vi "2D curvature tensor algebra.vi"(7 "2D tensor":T2, 9 "2D curvature Matrix IN":T1, 11 "curvature tensor IN":T3={"curvature Matrix"=[[3.0, 1.0], [1.0, 4.0]], "eigenvs"=[4.618033988749895, 2.381966011250105], "Eigenvectors"=[[-0.8506508083520399+0.0i, -0.5257311121191335+0.0i], [0.5257311121191335+0.0i, -0.8506508083520399+0.0i]], "theta (rad)"=0.5535743588970453, "theta (deg)"=31.717474411461012, "Δs"=[4.618033988749895, 2.381966011250105], "δG/G"=0.5535743588970453, "δs"=[4.618033988749895, 2.381966011250105], "inverse Matrix"=[[3.0, 1.0], [1.0, 4.0]], "noise T"=0.5535743588970453, "errors"={}} {"noise T" format="%#_3p"; "inverse Matrix" format="%#_3p"; "δs" format="%#_2p"; "δG/G" format="%#_3p"; "Δs" format="%#_3p"; "theta (deg)" format="%#_3p"; "curvature Matrix" format="%#_3p"; "eigenvs" format="%#_3p"; "Eigenvectors" format="%#_3p"; "theta (rad)" format="%#_3p"}) -> (1 "2D curvature Matrix OUT":T1, 3 "curvature tensor OUT":T3={"curvature Matrix"=[[3.0, 1.0], [1.0, 4.0]], "eigenvs"=[4.618033988749895, 2.381966011250105], "Eigenvectors"=[[-0.8506508083520399+0.0i, -0.5257311121191335+0.0i], [0.5257311121191335+0.0i, -0.8506508083520399+0.0i]], "theta (rad)"=0.5535743588970453, "theta (deg)"=31.717474411461012, "Δs"=[4.618033988749895, 2.381966011250105], "δG/G"=0.5535743588970453, "δs"=[4.618033988749895, 2.381966011250105], "inverse Matrix"=[[3.0, 1.0], [1.0, 4.0]], "noise T"=0.5535743588970453, "errors"={}} {"noise T" format="%#_3p"; "inverse Matrix" format="%#_3p"; "δs" format="%#_2p"; "δG/G" format="%#_3p"; "Δs" format="%#_3p"; "theta (deg)" format="%#_3p"; "curvature Matrix" format="%#_3p"; "eigenvs" format="%#_3p"; "Eigenvectors" format="%#_3p"; "theta (rad)" format="%#_3p"})   [LabVIEW 2020]
uses:
  2D curvature tensor.ctl
  <vilib>/Analysis/Matrix/Datatypes/RealMatrix.ctl
  <vilib>/Analysis/Matrix/Datatypes/ComplexMatrix.ctl
  3-lorentzian-parameters.ctl
  2D curvature tensor actions.ctl
  array of vectors -- algebra.ctl
  <vilib>/Analysis/baseanly.llb/Real Inverse Matrix.vi
  <vilib>/Analysis/7linalg.llb/Real Eigenvalues and Vectors.vi
  <vilib>/Analysis/NI_AALPro.lvlib
  <vilib>/Analysis/NI_AALBase.lvlib
  <vilib>/Analysis/Matrix/NI_Matrix.lvlib
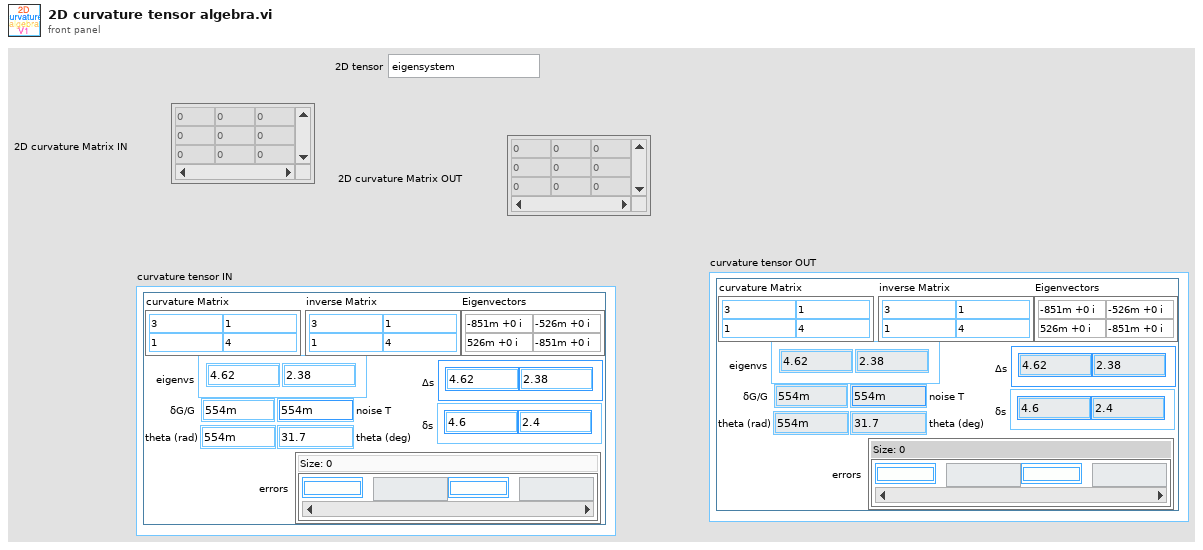
[diagram p1: front panel]
types:
  T1 = typedef "NI_Matrix.lvlib/RealMatrix.ctl" = dbl[][]
  T2 = typedef "2D curvature tensor actions.ctl" = enum16{"eigensystem", "sigma", "set matrix", "inverse"}
  T3 = typedef "2D curvature tensor.ctl" = cluster{"curvature Matrix":T1, "eigenvs":dbl[], "Eigenvectors":T4, "theta (rad)":dbl, "theta (deg)":dbl, "Δs":dbl[], "δG/G":dbl, "δs":dbl[], "inverse Matrix":T1, "noise T":dbl, "errors":map{T5, dbl}}
  T4 = typedef "NI_Matrix.lvlib/ComplexMatrix.ctl" = cdb[][]
  T5 = typedef "3-lorentzian-parameters.ctl" = enum16{"ζ", "τ1", "τS", "τN", "τC", "κ0", "m1", "m2", "m3", "T (K)", "B (T)", "θ (deg)", "side (S|R)", "set of (B|T)", "Re(offset)", "Im(offset)", "στ1", "στ1-", "στ1+", "στS", "στS-", "στS+"}
  T6 = typedef "array of vectors -- algebra.ctl" = enum16{"shift", "rotate", "scale", "multiply", "expectation"}
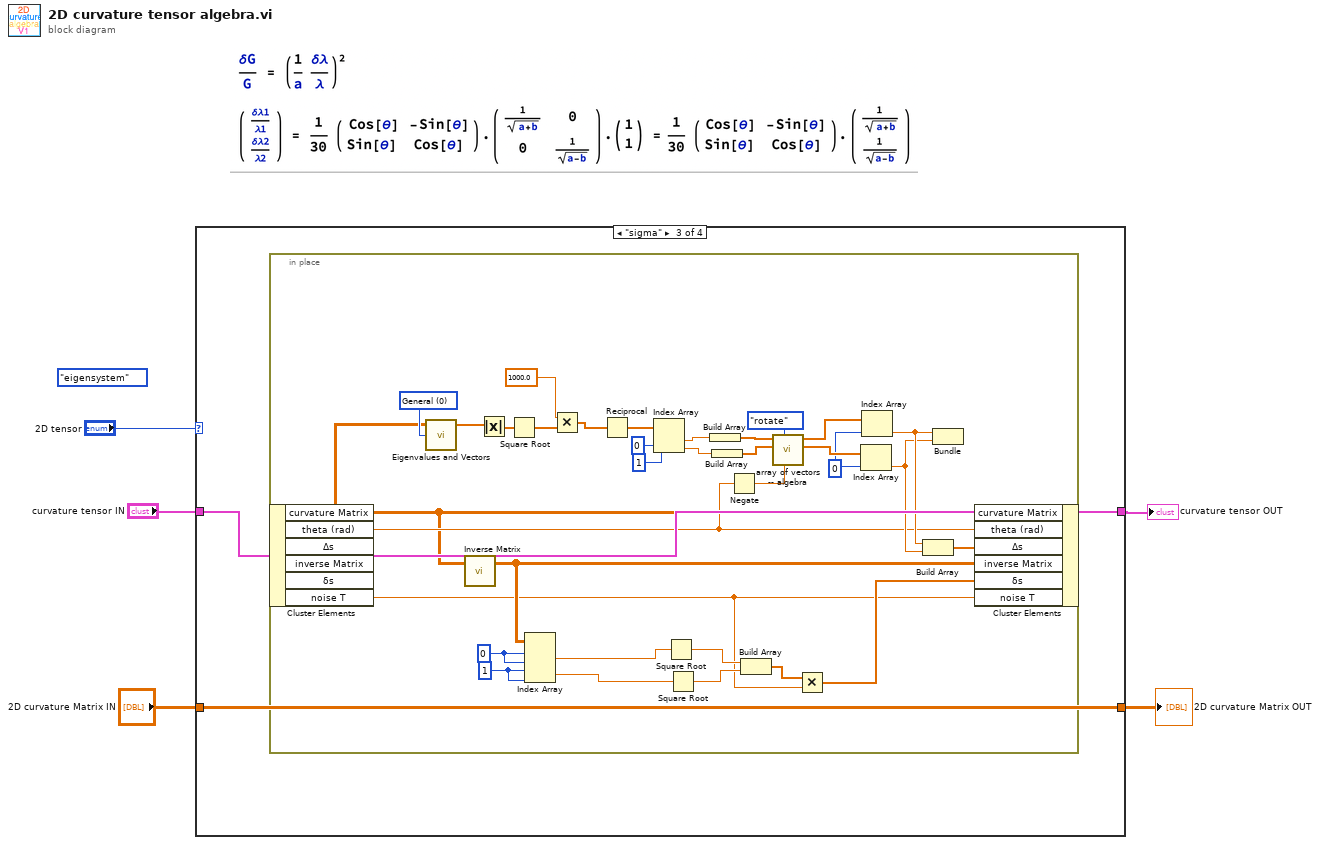
[diagram p0: block diagram]
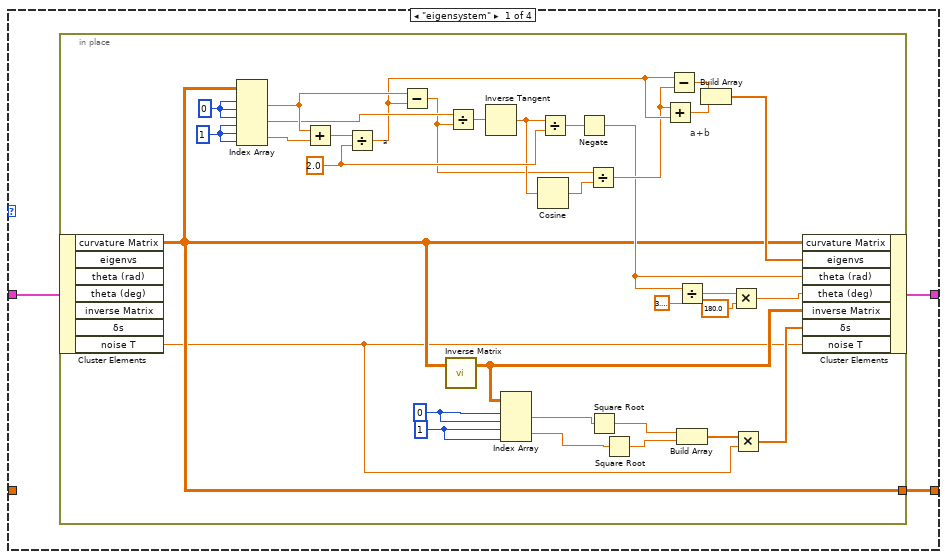
[diagram p2: hidden frame]
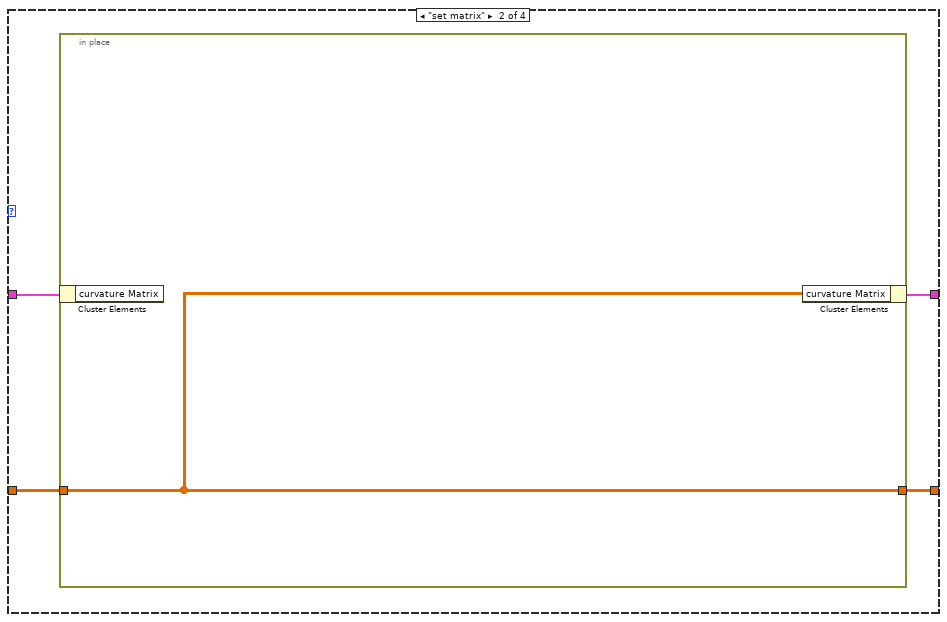
[diagram p3: hidden frame]
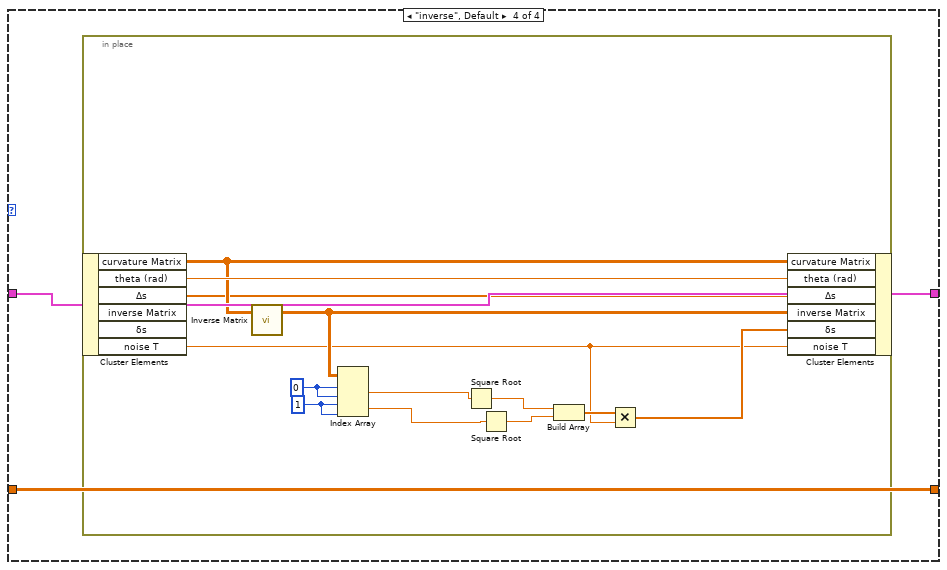
[diagram p4: hidden frame]
diagram:
  (unwired) 2D_curvature_tensor_actions."eigensystem" ("2D tensor")
  n1 = case shown="\"sigma\"" "2D tensor" {
    tunnel: [w7 w44 w47 w82] -> w4
    tunnel: "curvature tensor IN" -> [w8 w45 w47 w82]
    tunnel: [w6 w43 w48 w83] -> w2
    tunnel: "2D curvature Matrix IN" -> [_ w42 w48 w83]
    frame "eigensystem" {
      n2 = in-place {
        in-place-border: [w19] -> w6
        w14 = 1 ("index")
        w15 = 0 ("index")
        w35 = 2.0 ("y")
        w40 = 1 ("index (row)")
        w41 = 0 ("index (row)")
        # "a+b"
        # "a"
        n3 = in-place-cluster #1(w8) -> ("curvature Matrix"=w19:T1, "noise T"=w9:dbl)  [unwired: 5 out]
        n4 = Index Array(array=w19, index (row) #1=w41, index (col) #1=w41, index (row) #2=w41, index (col) #2=w40, index (row) #3=w40, index (col) #3=w40) -> (element #1=w37:dbl, element #2=w33:dbl, element #3=w39:dbl)
        n5 = Add(x=w37, y=w39) -> (x+y=w38:dbl)
        n6 = Divide(x=w38, y=w35) -> (x/y=w29:dbl)
        n7 = Subtract(x=w37, y=w29) -> (x-y=w31:dbl)
        n8 = call-poly <vilib>:"Inverse Matrix.vi"("Input Matrix"=w19) -> ("Inverse Matrix"=w11:T1)  [unwired: 1 in, 1 out]
        n9 = Divide(x=w33, y=w31) -> (x/y=w36:dbl)
        n10 = Inverse Tangent(1:w36) -> (0:w32:dbl)
        n11 = Index Array(array=w11, index (row) #1=w15, index (col) #1=w15, index (row) #2=w14, index (col) #2=w14) -> (element #1=w12:dbl, element #2=w13:dbl)
        n12 = Cosine(x=w32) -> (cos(x)=w30:dbl)
        n13 = Divide(x=w32, y=w35) -> (x/y=w34:dbl)
        n14 = Negate(x=w34) -> (-x=w22:dbl)
        n15 = Divide(x=w31, y=w30) -> (x/y=w28:dbl)
        n16 = Square Root ("Square Root.vi")(x=w12) -> (sqrt(x)=w18:dbl)
        n17 = Square Root ("Square Root.vi")(x=w13) -> (sqrt(x)=w17:dbl)
        n18 = Add(x=w28, y=w29) -> (x+y=w26:dbl)
        n19 = Subtract(x=w29, y=w28) -> (x-y=w27:dbl)
        n20 = Divide(x=w22, y=3.141592653589793) -> (x/y=w21:dbl)
        n21 = Build Array(w18, w17) -> (w16:dbl[])
        n22 = Build Array(w27, w26) -> (w25:dbl[])
        n23 = Multiply(x=w21, y=180.0) -> (x*y=w20:dbl)
        n24 = Multiply(x=w16, y=w9) -> (x*y=w10:dbl[])
        n25 = in-place-cluster #1("curvature Matrix"=w19, "eigenvs"=w25, "theta (rad)"=w22, "theta (deg)"=w20, "inverse Matrix"=w11, "δs"=w10, "noise T"=w9) -> (w7:T3)
      }
    }
    frame "set matrix" {
      n26 = in-place {
        in-place-border: [w46] -> w43
        in-place-border: w42 -> [w46]
        n27 = in-place-cluster #2(w45) -> ()  [unwired: 1 out]
        n28 = in-place-cluster #2("curvature Matrix"=w46) -> (w44:T3)
      }
    }
    frame "sigma" {
      n29 = in-place {
        w53 = 1 ("index")
        w54 = 0 ("index")
        w66 = 0 ("index")
        w76 = 0 items=["General", "Symmetric"] ("matrix type")
        n30 = in-place-cluster #3(w47) -> ("curvature Matrix"=w59:T1, "theta (rad)"=w60:dbl, "noise T"=w49:dbl)  [unwired: 3 out]
        n31 = call-poly <vilib>:"Eigenvalues and Vectors.vi"("matrix type"=w76, "Input Matrix"=w59) -> ("Eigenvalues"=w75:cdb[])  [unwired: 1 in, 2 out]
        n32 = call-poly <vilib>:"Inverse Matrix.vi"("Input Matrix"=w59) -> ("Inverse Matrix"=w55:T1)  [unwired: 1 in, 1 out]
        n33 = Absolute Value(x=w75) -> (abs(x)=w81:dbl[])
        n34 = Square Root ("Square Root.vi")(x=w81) -> (sqrt(x)=w78:dbl[])
        n35 = Index Array(array=w55, index (row) #1=w54, index (col) #1=w54, index (row) #2=w53, index (col) #2=w53) -> (element #1=w51:dbl, element #2=w52:dbl)
        n36 = Multiply(x=1000.0, y=w78) -> (x*y=w65:dbl[])
        n37 = Reciprocal(x=w65) -> (1/x=w77:dbl[])
        n38 = Index Array(array=w77, index #1=0 ("index"), index #2=1 ("index")) -> (element #1=w74:dbl, element #2=w73:dbl)
        n39 = Square Root ("Square Root.vi")(x=w51) -> (sqrt(x)=w58:dbl)
        n40 = Square Root ("Square Root.vi")(x=w52) -> (sqrt(x)=w57:dbl)
        n41 = Build Array(w74) -> (w71:dbl[])
        n42 = Build Array(w73) -> (w70:dbl[])
        n43 = Negate(x=w60) -> (-x=w72:dbl)
        n44 = Build Array(w58, w57) -> (w56:dbl[])
        n45 = call "array of vectors -- algebra.vi"("theta"=w72, "Enum"=array_of_vectors_--_algebra."rotate", "y IN"=w70, "x IN"=w71) -> ("y IOUT"=w67:dbl[], "x  OUT"=w68:dbl[])  [unwired: 5 in, 1 out]
        n46 = Multiply(x=w56, y=w49) -> (x*y=w50:dbl[])
        n47 = Index Array(array=w67, index=w66) -> (element=w62:dbl)
        n48 = Index Array(array=w68, index=w66) -> (element=w63:dbl)
        n49 = Build Array(w63, w62) -> (w61:dbl[])
        n50 = Bundle("Numeric"=w63, "Numeric"=w62) -> ()  [unwired: 1 in, 1 out]
        n51 = in-place-cluster #3("curvature Matrix"=w59, "theta (rad)"=w60, "Δs"=w61, "inverse Matrix"=w55, "δs"=w50, "noise T"=w49) -> ()  [unwired: 1 out]
      }
    }
    frame "inverse", Default {
      n52 = in-place {
        w89 = 1 ("index")
        w90 = 0 ("index")
        n53 = in-place-cluster #4(w82) -> ("curvature Matrix"=w95:T1, "theta (rad)"=w96:dbl, "Δs"=w86:dbl[], "noise T"=w84:dbl)  [unwired: 2 out]
        n54 = call-poly <vilib>:"Inverse Matrix.vi"("Input Matrix"=w95) -> ("Inverse Matrix"=w91:T1)  [unwired: 1 in, 1 out]
        n55 = Index Array(array=w91, index (row) #1=w90, index (col) #1=w90, index (row) #2=w89, index (col) #2=w89) -> (element #1=w87:dbl, element #2=w88:dbl)
        n56 = Square Root ("Square Root.vi")(x=w87) -> (sqrt(x)=w94:dbl)
        n57 = Square Root ("Square Root.vi")(x=w88) -> (sqrt(x)=w93:dbl)
        n58 = Build Array(w94, w93) -> (w92:dbl[])
        n59 = Multiply(x=w92, y=w84) -> (x*y=w85:dbl[])
        n60 = in-place-cluster #4("curvature Matrix"=w95, "theta (rad)"=w96, "Δs"=w86, "inverse Matrix"=w91, "δs"=w85, "noise T"=w84) -> ()  [unwired: 1 out]
      }
    }
  }
  "curvature tensor OUT" <- w4
  "2D curvature Matrix OUT" <- w2
